vi "DATA DIGITAL.vi"(8 "error in":errorcluster, 10 "DIGITAL DAQ":bool[](array[boolean])) -> (0 "error out":errorcluster)   [LabVIEW 2020]
doc: "LOS DATOS DE DIGITAL\n_____\nCreated using Delacor QMH Event Scripter 6.0.0.121."
uses:
  DATA DIGITAL Argument--cluster.ctl
  Acquisition.lvlib
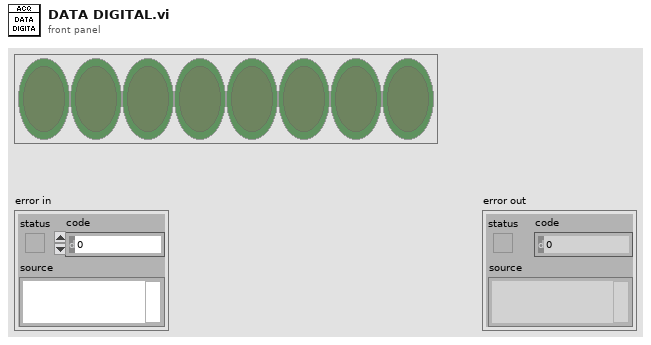
[diagram p1: front panel]
types:
  T1 = typedef "DATA DIGITAL Argument--cluster.ctl" = cluster{"DIGITAL DAQ":bool[]}
  T2 = typedef "Acquisition.lvlib/Request Events--cluster.ctl" = cluster{"Stop Module":refnum<user-event>, "Show Panel":refnum<user-event>, "Hide Panel":refnum<user-event>, "Get Module Execution Status":refnum<user-event>, "Show Diagram":refnum<user-event>, "Start Acquisition":refnum<user-event>, "Configurar tarea Analogico":refnum<user-event>, "Configurar Tarea Digital":refnum<user-event>, "Wake up Helper loop Analogico":refnum<user-event>, "Wake up HL digital":refnum<user-event>, "STOP HL ANALOGICO":refnum<user-event>, "STOP HL DIGITAL":refnum<user-event>}
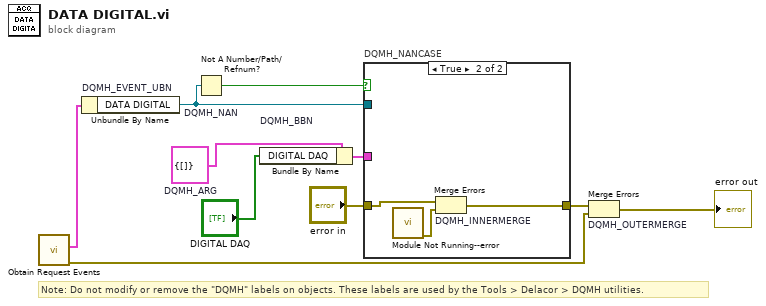
[diagram p0: block diagram]
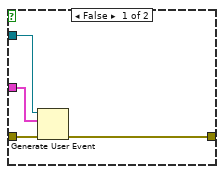
[diagram p2: hidden frame]
diagram:
  w4 = T1 {"DIGITAL DAQ"=[]}  # DQMH_ARG
  # "Note: Do not modify or remove the \"DQMH\" labels on objects. These labels are used by the Tools > Delacor > DQMH utilities."
  n1 = call "Obtain Request Events.vi"() -> ("error out"=w2:errorcluster, "Acquisition Request Events"=w1:T2)  [unwired: 10 in]
  n2 = Unbundle By Name "DQMH_EVENT_UBN"(w1) -> ("DATA DIGITAL"=w6:refnum<user-event>)
  n3 = Not A Number/Path/Refnum? "DQMH_NAN"(number/path/refnum=w6) -> (NaN/Path/Refnum?=w7:bool)
  n4 = Bundle By Name "DQMH_BBN"(cluster=w4, "DIGITAL DAQ"="DIGITAL DAQ") -> (w8:T1)
  n5 = case "DQMH_NANCASE" shown="True" w7 {
    tunnel: "error in" -> [w14 w17]
    tunnel: [w13 w16] -> w5
    tunnel: w6 -> [w12 _]
    tunnel: w8 -> [w11 _]
    frame False {
      n6 = Generate User Event(user event=w12, event data cluster=w11, error in=w14) -> (error out=w13:errorcluster)  [unwired: 1 in, 1 out]
    }
    frame True {
      n7 = call "Module Not Running--error.vi"() -> ("error out"=w15:errorcluster)  [unwired: 11 in]
      n8 = Merge Errors "DQMH_INNERMERGE"(w17, w15) -> (w16:errorcluster)
    }
  }
  n9 = Merge Errors "DQMH_OUTERMERGE"(w5, w2) -> (→"error out":errorcluster)
